vi "KeithleyMeter Control Panel.vi"(8 "error in (no error)":errorcluster, 11 "Class":refnum<class "KeithleyMeter.lvclass">) -> (0 "error out":errorcluster, 3 "KeithleyMeter out":refnum<class "KeithleyMeter.lvclass">)   [LabVIEW 2015, in "KeithleyMeter.lvclass"]
uses:
  KeithleyMeter.lvclass
  KeithleyMeter Data.ctl
  KeithleyMeter Function.ctl
panel:
  in  "Data":T1={"Range (-1: auto)"=20.0, "Integration Time (NPLCs)"=1.0, "Function"=enum."VOLTAGE", "W Offset comp"=TRUE, "4-wire W"=TRUE} {"Integration Time (NPLCs)" min=0.01 max=10.0 step=0.01 format="%.2f"}
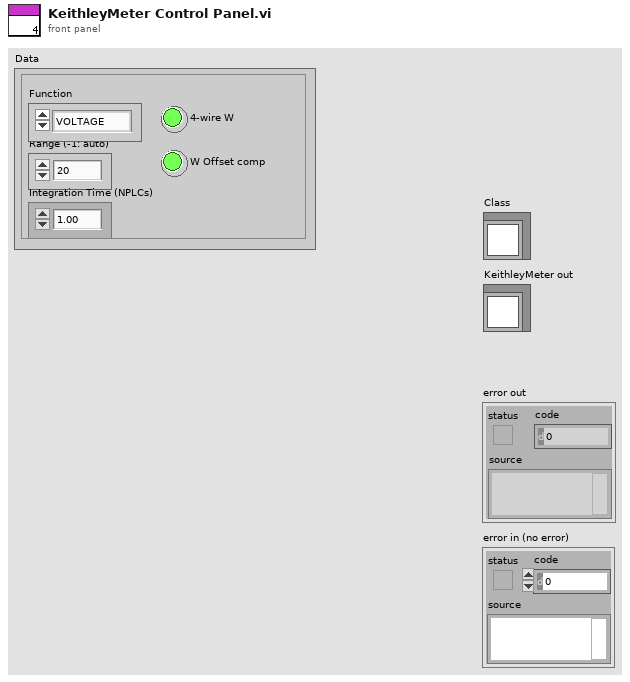
[diagram p1: front panel]
types:
  T1 = typedef "KeithleyMeter Data.ctl" = cluster{"Range (-1: auto)":dbl, "Integration Time (NPLCs)":dbl, "Function":T2, "W Offset comp":bool, "4-wire W":bool}
  T2 = typedef "KeithleyMeter Function.ctl" = enum16{"VOLTAGE", "CURRENT", "RESISTANCE"}
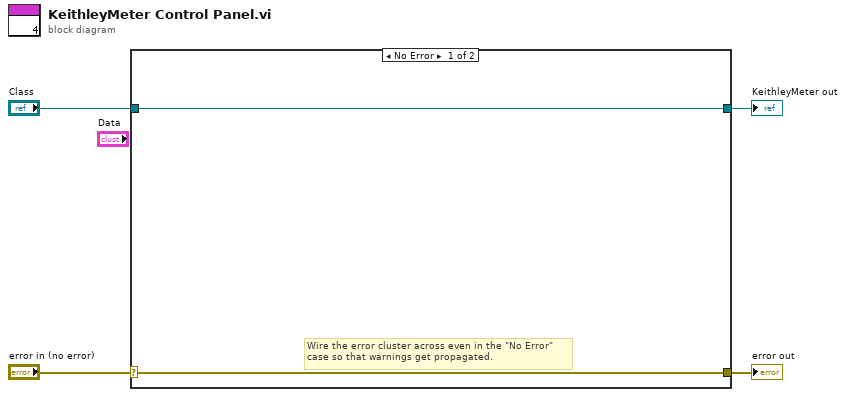
[diagram p0: block diagram]
diagram:
  n1 = case shown="No Error" "error in (no error)" {
    selector: "error in (no error)" -> [w5 w8]
    tunnel: [w5 w8] -> w3
    tunnel: [w6 w7] -> w1
    tunnel: "Class" -> [w6 w7]
    frame No Error {
      # "Wire the error cluster across even in the \"No Error\"\ncase so that warnings get propagated."
    }
    frame Error {
    }
  }
  "error out" <- w3
  "KeithleyMeter out" <- w1
